vi "SGDA-Globals.vi"() -> ()   [LabVIEW 2020]
uses:
  Type Defs/Hardware Destination.ctl
panel:
  in  "Hardware":T1=enum."PXI"
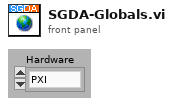
[diagram p1: front panel]
types:
  T1 = typedef "Hardware Destination.ctl" = enum16{"None", "PXI", "TDT", "NI", "TDTSIM"}
diagram:
